vi "Lab_3.vi"() -> ()   [LabVIEW 2025]
uses:
  Runner_Data_Structure.ctl
  HR_Data_Structure.ctl
  Raw_Data_IN_HR.ctl
panel:
  in  "File Path":path
  in  "Runner's Data":T1
  out "Error OUT":errorcluster
  in  "Error IN":errorcluster
  out "BPM":cluster{"Time":timestamp[], "Bpm":i32[]}(graph)
  out "Zone PLOT":T2(graph)
  out "Zone Data":string[][](array[string]) caption="HEART RATE ZONES"
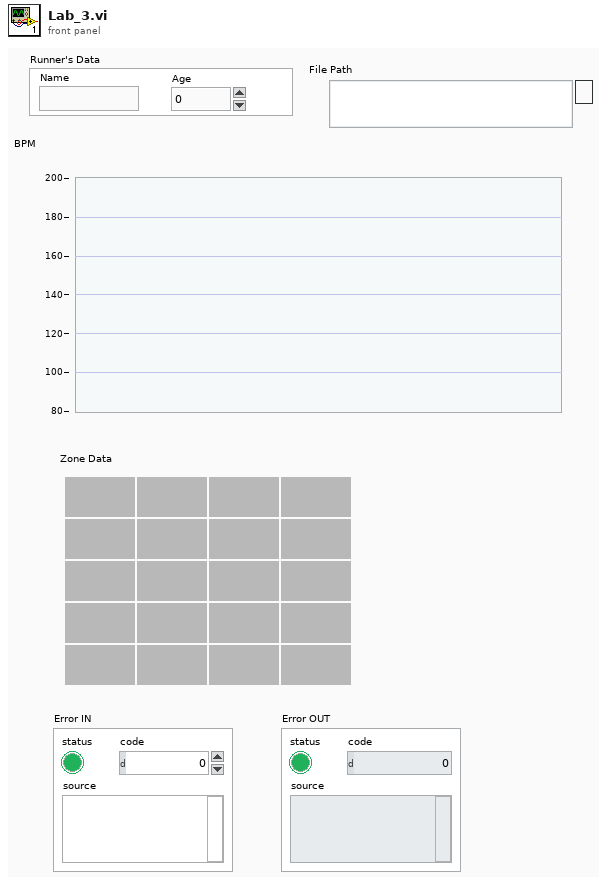
[diagram p1: front panel]
types:
  T1 = typedef "Runner_Data_Structure.ctl" = cluster{"Name":string, "Age":i32}
  T2 = cluster{"Total Time in Zone":dbl[], "Heart Rate Zone No":dbl[]}
  T3 = typedef "HR_Data_Structure.ctl" = cluster{"HR Max":i32, "% HR MAX ":dbl[], "Raw Data":T4, "Runner's Data":T1, "HR Zone":string[][], "Total Time in Zone":dbl[], "Heart Rate Zone No":dbl[]}
  T4 = typedef "Raw_Data_IN_HR.ctl" = cluster{"Time":timestamp[], "Bpm":i32[]}
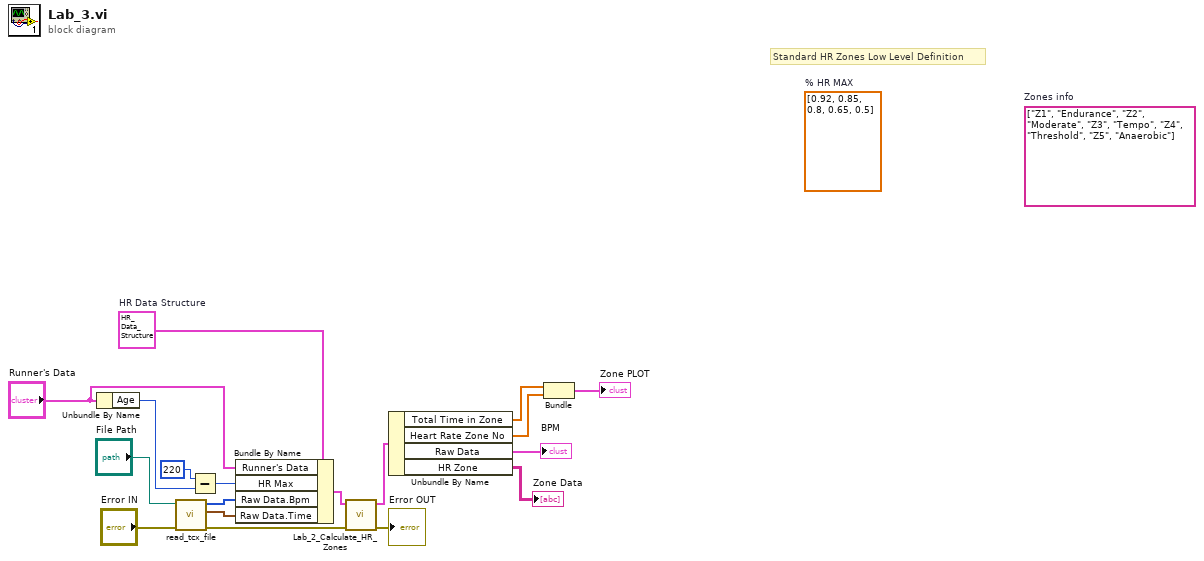
[diagram p0: block diagram]
diagram:
  w18 = T3 data[18004B]  # HR Data Structure
  (unwired) string[][] [["Z1", "Endurance"], ["Z2", "Moderate"], ["Z3", "Tempo"], ["Z4", "Threshold"], ["Z5", "Anaerobic"]]  # Zones info
  (unwired) dbl[] [0.92, 0.85, 0.8, 0.65, 0.5]  # % HR MAX
  # "Standard HR Zones Low Level Definition"
  n1 = Unbundle By Name("Runner's Data") -> ("Age"=w15:i32)
  n2 = call "read_tcx_file.vi"("error in"="Error IN", "File Path"="File Path") -> ("error out"=w8:errorcluster, "Time"=w10:timestamp[], "Bmp"=w11:i32[])  [unwired: 7 in]
  n3 = Subtract(x=220, y=w15) -> (x-y=w14:i32)
  n4 = Bundle By Name(cluster=w18, "Runner's Data"="Runner's Data", "HR Max"=w14, "Raw Data.Bpm"=w11, "Raw Data.Time"=w10) -> (w9:T3)
  n5 = call "Lab_2_Calculate_HR_Zones.vi"("Error IN"=w8, "HR Data Structure IN"=w9) -> ("Error OUT"=→"Error OUT":errorcluster, "HR Data Structure OUT"=w6:T3)  [unwired: 8 in]
  n6 = Unbundle By Name(w6) -> ("Total Time in Zone"=w3:dbl[], "Heart Rate Zone No"=w4:dbl[], "Raw Data"=→"BPM":T4, "HR Zone"=→"Zone Data":string[][])
  n7 = Bundle("Total Time in Zone"=w3, "Heart Rate Zone No"=w4) -> (→"Zone PLOT":T2)  [unwired: 1 in]
